vi "VI Tester Project API Open VI Tester.vi"(8 "error in":errorcluster, 11 "Object":T1) -> (0 "error out":errorcluster)   [LabVIEW 2013]
uses:
  VITester Project Item Ref.ctl
  VI Tester Project API Method Selector - Enum.ctl
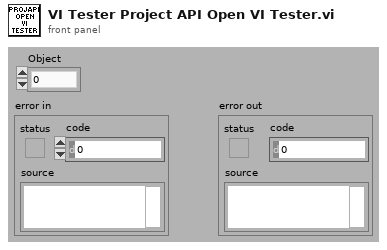
[diagram p1: front panel]
types:
  T1 = typedef "VITester Project Item Ref.ctl" = u64
  T2 = typedef "VI Tester Project API Method Selector - Enum.ctl" = enum16{"Open VI Tester", "Run All Tests", "Create New TestCase", "Create New TestSuite"}
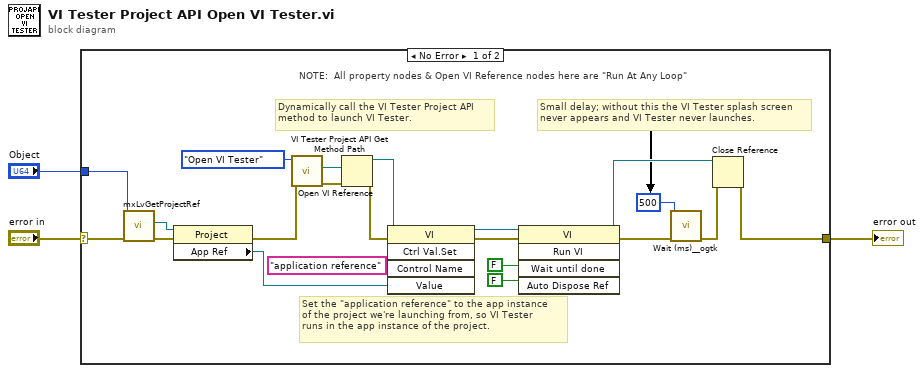
[diagram p0: block diagram]
diagram:
  n1 = case shown="No Error" "error in" {
    selector: "error in" -> [w11 w25]
    tunnel: [w24 w25] -> w3
    tunnel: "Object" -> [w21 _]
    frame No Error {
      # "Set the \"application reference\" to the app instance\nof the project we're launching from, so VI Tester\nruns in the app instance of the project."
      # "Dynamically call the VI Tester Project API\nmethod to launch VI Tester."
      # "Small delay; without this the VI Tester splash screen\nnever appears and VI Tester never launches."
      # "NOTE:  All property nodes & Open VI Reference nodes here are \"Run At Any Loop\""
      n2 = call <resource>:"mxLvGetProjectRef.vi"("error in"=w11, "Item"=w21) -> ("error out"=w12:errorcluster, "Project Refnum"=w13:refnum<vi>)  [unwired: 7 in, 1 out]
      n3 = property class="Project"(reference=w13, error in=w12) -> (error out=w6:errorcluster, "App Ref"=w7:refnum<vi>)  [unwired: 1 out]
      n4 = call "VI Tester Project API Get Method Path.vi"("error in (no error)"=w6, "Project API Method"=VI_Tester_Project_API_Method_Selector_-_Enum."Open VI Tester") -> ("error out"=w9:errorcluster, "Path to VI Tester Project API Proxy VI"=w22:path)  [unwired: 8 in]
      n5 = Open VI Reference(vi path=w22, error in (no error)=w9) -> (vi reference=w5:refnum<vi>, error out=w17:errorcluster)  [unwired: 4 in]
      n6 = invoke class="VI" method="Ctrl Val.Set"(reference=w5, error in=w17, "Control Name"="application reference", "Value"=w7) -> (reference out=w15:refnum<vi>, error out=w16:errorcluster)  [unwired: 1 in, 3 out]
      n7 = invoke class="VI" method="Run VI"(reference=w15, error in=w16, "Wait until done"=FALSE ("Wait Until Done"), "Auto Dispose Ref"=FALSE ("Auto Dispose Reference")) -> (reference out=w8:refnum<vi>, error out=w18:errorcluster)  [unwired: 1 in, 3 out]
      n8 = call <userlib>:"Wait (ms)__ogtk.vi"("error in (no error)"=w18, "milliseconds to wait"=u32 500) -> ("error out"=w23:errorcluster)  [unwired: 8 in, 1 out]
      n9 = Close Reference(reference=w8, error in (no error)=w23) -> (error out=w24:errorcluster)
    }
    frame Error {
    }
  }
  "error out" <- w3
